vi "HD3000.vi"() -> ()   [LabVIEW 2013]
uses:
  <vilib>/vision/NI_Vision_Development_Module.lvlib
  <vilib>/ptbypt/NI_PtbyPt.lvlib
panel:
  out "Numeric 3":i32
  out "Numeric 2":i32
  out "Numeric":i32
  out "Done":bool caption="Stopped"
  out "error out 4":errorcluster
  out "error out 3":errorcluster
  out "error out 2":errorcluster
  out "Mean Value":sgl
  out "Frame Rate":dbl
  in  "Display":bool
  in  "Rec":bool
  in  "Start":bool
  in  "?":enum32{"Settings", "Monitor", "Errors"}(tab)
  in  "Selected Path for AVI":path
  in  "Cluster":T1={"Brightness"=133, "Contrast"=0.05, "Saturation"=83, "Sharpness"=25, "White Balance"=3040, "Exposure"=0.00048828125, "Auto"=FALSE, "Auto"=FALSE} {"Exposure" min=0.00048828125 max=2.0 scale=0.00048828125..2.0 scale format="%#_1f"; "White Balance" min=2800 max=8000 step=1 scale=2800.0..10000.0; "Sharpness" min=0 max=50 step=1 scale=0.0..50.0; "Saturation" min=0 max=200 step=1 scale=0.0..200.0; "Contrast" min=0.0 max=0.1 scale=0.0..0.1; "Brightness" min=30 max=255 step=1 scale=30.0..255.0}
  out "Rec Time":dbl format="%#_3g"
  out "Est. fps":dbl format="%#_2g"
  out "Frames Recorded":dbl
  out "Frames not Recorded":dbl
  out "Image Number":u32
  out "Lost Image Count":u32
  out "Total Images Transferred":u32
  in  "Interface Name":string="cam1"
  out "error out":errorcluster
  out "Histogram":T2(graph)
  out "Image":T3(plugin-control)
  in  "Stop (F)":bool
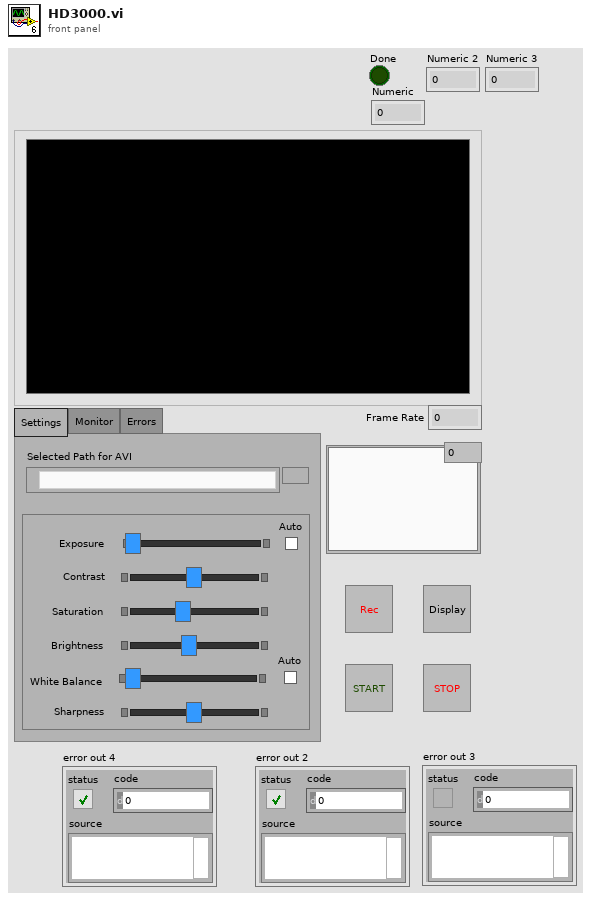
[diagram p1: front panel]
types:
  T1 = cluster{"Brightness":i64, "Contrast":dbl, "Saturation":i64, "Sharpness":i64, "White Balance":i64, "Exposure":dbl, "Auto":bool, "Auto":bool}
  T2 = cluster{"Starting Value":sgl, "Incremental Value":sgl, "Histogram":u32[]}
  T3 = typedef "IMAQ Image.ctl" = refnum<image>
  T4 = typedef "Image Type" = u32
  T5 = typedef "AviRefnum.ctl" = refnum<k1>
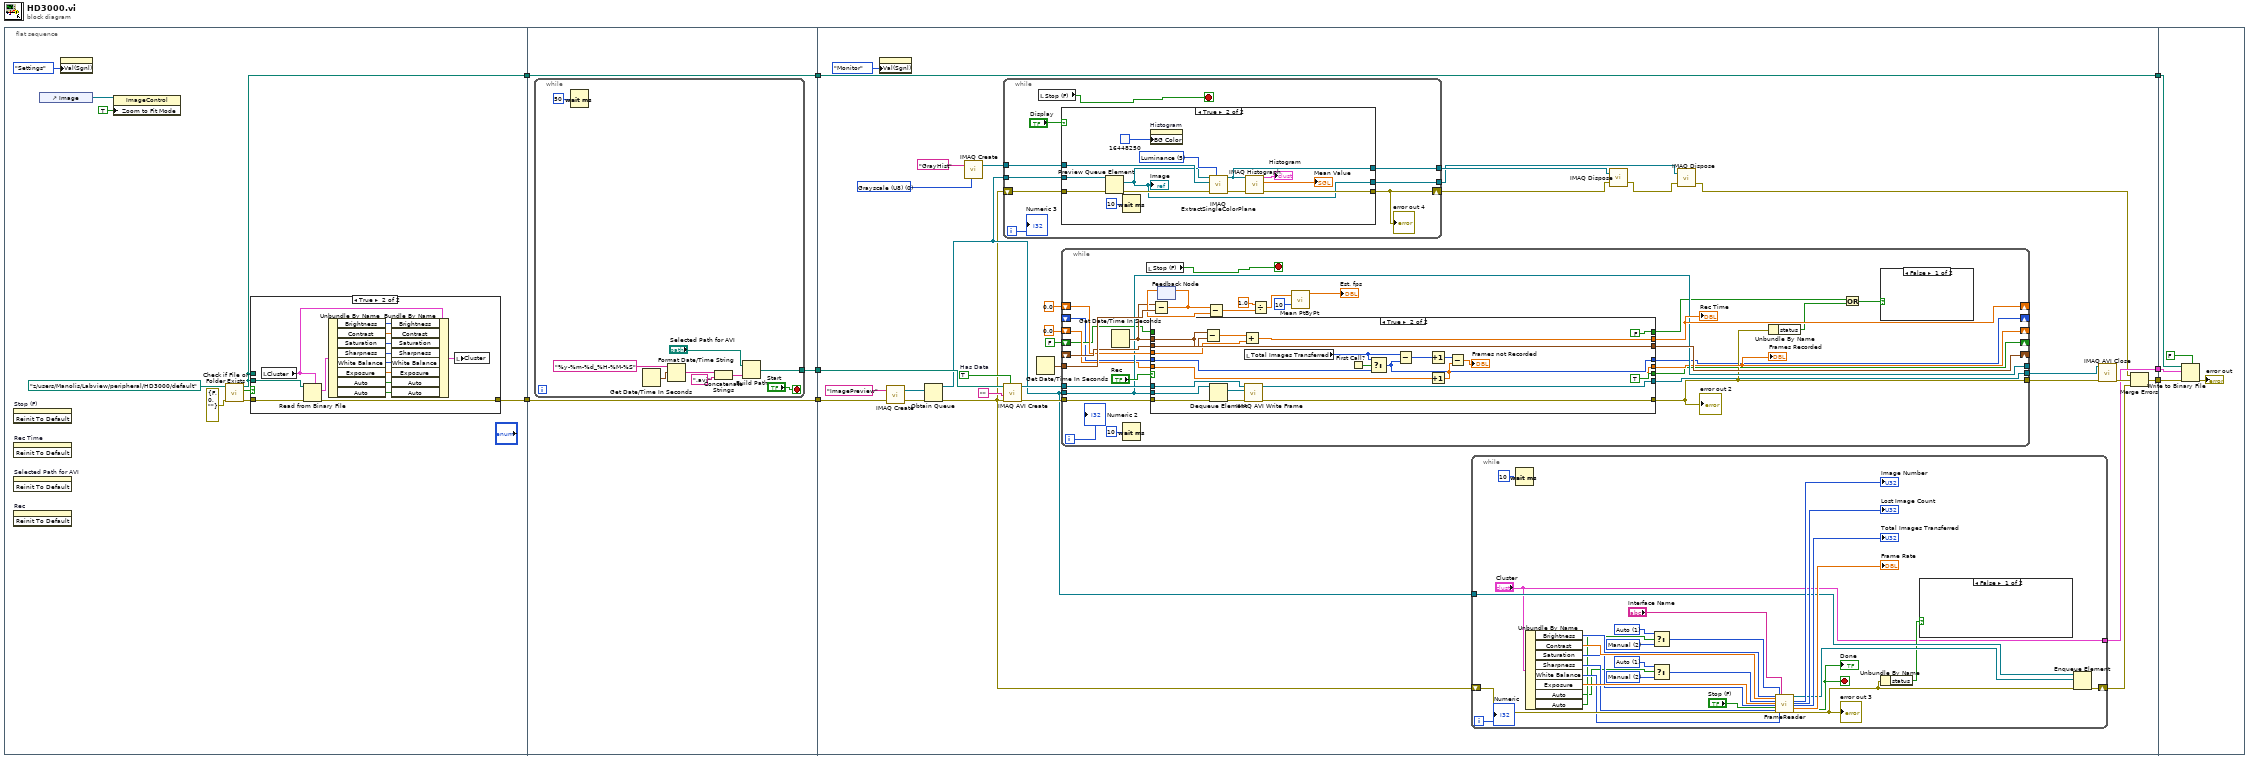
[diagram p0: block diagram]
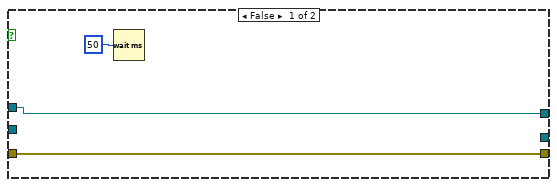
[diagram p3: hidden frame]
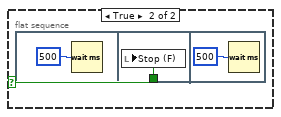
[diagram p4: hidden frame]
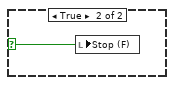
[diagram p5: hidden frame]
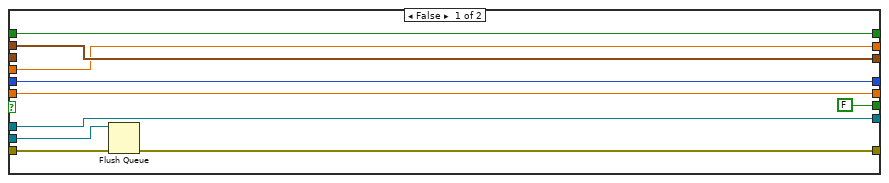
[diagram p6: hidden frame]
diagram:
  n1 = flat-sequence {
    tunnel: [w12] -> w6
    tunnel: [w9] -> w1
    tunnel: [w35] -> w8
    tunnel: w6 -> [w34]
    tunnel: [w34] -> w5
    tunnel: [w33] -> w2
    tunnel: w1 -> [w33]
    tunnel: w8 -> [w71]
    tunnel: [w50] -> w7
    tunnel: w5 -> [w55]
    tunnel: [w55] -> w4
    tunnel: [w54] -> w3
    tunnel: w2 -> [w53]
    tunnel: w7 -> [w204]
    tunnel: w4 -> [w202]
    tunnel: w3 -> [w200]
    frame #0 {
      n2 = invoke on="Stop (F)" class="Bool (strict)" method="Reinit To Default"() -> ()  [unwired: 3 in, 3 out]
      n3 = invoke on="Rec Time" class="DigNum (strict)" method="Reinit To Default"() -> ()  [unwired: 3 in, 3 out]
      n4 = invoke on="Selected Path for AVI" class="Path" method="Reinit To Default"() -> ()  [unwired: 3 in, 3 out]
      n5 = invoke on="Rec" class="Bool (strict)" method="Reinit To Default"() -> ()  [unwired: 3 in, 3 out]
      n6 = control-ref of="Image"() -> (w15:refnum<vi>)
      n7 = property class="TabCtl (strict)"("Val(Sgnl)"=enum32{"Settings", "Monitor"}."Settings" ("Value (Signaling)")) -> ()  [unwired: 2 in, 2 out]
      n8 = property on="Property Node" class="ImageControl"(reference=w15, "Zoom to Fit Mode"=TRUE) -> ()  [unwired: 1 in, 2 out]
      n9 = call <vilib>:"Check if File or Folder Exists.vi"("error in (no error)"=errorcluster {"status"=FALSE, "code"=0, "source"=""} ("error in"), "path"=path "z:/users/Manolis/Labview/peripheral/HD3000/default" ("file path")) -> ("error out"=w10:errorcluster, "file or folder exists?"=w13:bool, "dup path"=w12:path)  [unwired: 7 in]
      n10 = case shown="True" w13 {
        tunnel: w12 -> [_ w23]
        tunnel: w12 -> [_ _]
        tunnel: w10 -> [w18 w22]
        tunnel: [w18 w21] -> w9
        frame False {
        }
        frame True {
          n11 = local read "Cluster"() -> (w20:T1)
          n12 = Read from Binary File(5:w20, 8:w22, 11:w23) -> (0:w21:errorcluster, 2:w32:T1)  [unwired: 3 in, 2 out]
          n13 = Unbundle By Name(w32) -> ("Brightness"=w31:i64, "Contrast"=w30:dbl, "Saturation"=w29:i64, "Sharpness"=w28:i64, "White Balance"=w27:i64, "Exposure"=w26:dbl, "Auto"=w25:bool, "Auto"=w24:bool)
          n14 = Bundle By Name(cluster=w20, "Brightness"=w31, "Contrast"=w30, "Saturation"=w29, "Sharpness"=w28, "White Balance"=w27, "Exposure"=w26, "Auto"=w25, "Auto"=w24) -> (w19:T1)
          n15 = local write "Cluster"(w19) -> ()
        }
      }
    }
    frame #1 {
      n16 = while {
        tunnel: [w36] -> w35
        stop <- "Start" stop-if-true
        n17 = Wait (ms)(milliseconds to wait=u32 50) -> ()  [unwired: 1 out]
        n18 = Get Date/Time In Seconds() -> (seconds since 1Jan1904=w42:timestamp)
        n19 = Format Date/Time String(time format string (%c)="%y-%m-%d_%H-%M-%S", seconds (now)=w42) -> (date/time string=w40:string)  [unwired: 1 in]
        n20 = Concatenate Strings(w40, ".avi" ("search string")) -> (w38:string)
        n21 = Build Path(base path="Selected Path for AVI", name or relative path=w38) -> (appended path=w36:path)
      }
    }
    frame #2 {
      w65 = T4 0 items=["Grayscale (U8)", "Grayscale (I16)", "Grayscale (SGL)", "Complex (CSG)", "RGB (U32)", "HSL (U32)", "RGB (U64)", "Grayscale (U16)"] ("Image Type")
      w67 = TRUE  # Has Data
      n22 = property class="TabCtl (strict)"("Val(Sgnl)"=enum32{"Settings", "Monitor"}."Monitor" ("Value (Signaling)")) -> ()  [unwired: 2 in, 2 out]
      n23 = call "IMAQ Create"("Image Name"="ImagePreview", "error in (no error)"=w53) -> ("New Image"=w61:T3, "error out"=w52:errorcluster)  [unwired: 3 in]
      n24 = Obtain Queue(element data type=w61, error in (no error)=w52) -> (queue out=w60:refnum<queue>, error out=w51:errorcluster)  [unwired: 3 in, 1 out]
      n25 = call "IMAQ Create"("Image Name"="GrayHist", "Image Type"=w65) -> ("New Image"=w63:T3)  [unwired: 3 in, 1 out]
      n26 = while {
        tunnel: w60 -> [w83]
        tunnel: w63 -> [w84]
        shift-right: [w81] -> w48
        shift-left: w51 -> [w80]
        tunnel: [w78] -> w49
        tunnel: [w77] -> w45
        i -> [w79]
        stop <- w76 stop-if-true
        n27 = local read "Stop (F)"() -> (w76:bool)
        n28 = case shown="True" "Display" {
          tunnel: w84 -> [w85 w97]
          tunnel: w83 -> [_ w95]
          tunnel: [w86 w93] -> w81
          tunnel: w80 -> [w86 w92]
          tunnel: [w85 w89] -> w78
          tunnel: [_ w88] -> w77
          frame False {
            n29 = Wait (ms)(milliseconds to wait=u32 50) -> ()  [unwired: 1 out]
          }
          frame True {
            w99 = 5 items=["Red", "Green", "Blue", "Hue", "Saturation", "Luminance", "Value", "Intensity"] ("Color Plane")
            n30 = Preview Queue Element(queue=w95, error in (no error)=w92) -> (element=w88:T3, error out=w91:errorcluster)  [unwired: 1 in, 2 out]
            "Image" <- w88
            n31 = Wait (ms)(milliseconds to wait=u32 10) -> ()  [unwired: 1 out]
            n32 = property on="Histogram" class="WFGraph (strict)"("BG Color"=u32 16448250) -> ()  [unwired: 2 in, 2 out]
            n33 = call "IMAQ ExtractSingleColorPlane"("Color Plane"=w99, "error in (no error)"=w91, "Image Dst"=w97, "Image Src"=w88) -> ("error out"=w94:errorcluster, "Image Dst Out"=w89:T3)  [unwired: 6 in]
            n34 = call "IMAQ Histograph"("error in (no error)"=w94, "Image"=w89) -> ("error out"=w93:errorcluster, "Mean Value"=→"Mean Value":sgl, "Histogram Graph"=→"Histogram":T2)  [unwired: 6 in, 1 out]
          }
        }
        "error out 4" <- w81
        "Numeric 3" <- w79
      }
      n35 = call "IMAQ AVI Create"("Has Data"=w67, "error in (no error)"=w51, "Compression Filter"="", "AVI Path"=w71) -> ("error out"=w72:errorcluster, "Avi Refnum"=w75:T5)  [unwired: 3 in, 3 out]
      n36 = Get Date/Time In Seconds() -> (seconds since 1Jan1904=w69:timestamp)
      n37 = while {
        tunnel: [w165] -> w74
        tunnel: [w145] -> w73
        tunnel: w75 -> [w164]
        tunnel: w72 -> [w163]
        tunnel: w69 -> [w162]
        shift-right: [w161] -> _
        shift-left: _ -> [w160]
        shift-right: [w158] -> _
        shift-left: 0.0 -> [w159]
        tunnel: [w148] -> _
        tunnel: w60 -> [w148]
        shift-right: [w147] -> _
        shift-left: 0.0 -> [w146]
        shift-right: [w144] -> _
        shift-left: FALSE ("First Call?: T/F") -> [w143]
        shift-right: [w140] -> _
        shift-left: _ -> [w139]
        i -> [w136]
        stop <- w135 stop-if-true
        n38 = Get Date/Time In Seconds() -> (seconds since 1Jan1904=w152:timestamp)
        n39 = Wait (ms)(milliseconds to wait=u32 10) -> ()  [unwired: 1 out]
        n40 = local read "Stop (F)"() -> (w135:bool)
        n41 = case shown="True" "Rec" {
          tunnel: [w176 w199] -> w165
          tunnel: [w167 w198] -> w145
          tunnel: w164 -> [w176 w197]
          tunnel: w163 -> [w168 w188]
          tunnel: [w174 w192] -> w158
          tunnel: [w175 w195] -> w161
          tunnel: w152 -> [w175 w195]
          tunnel: w160 -> [_ w194]
          tunnel: w159 -> [w174 w193]
          tunnel: w148 -> [w173 w191]
          tunnel: [w172 w178] -> w147
          tunnel: w146 -> [w172 w189]
          tunnel: [FALSE ("First Call?: T/F") TRUE ("First Call?: T/F")] -> w144
          tunnel: w143 -> [w171 _]
          tunnel: [w171 FALSE ("First Call?: T/F")] -> w142
          tunnel: [w169 w182] -> w140
          tunnel: w139 -> [w169 w183]
          frame False {
            n42 = Flush Queue(queue=w173, error in (no error)=w168) -> (error out=w167:errorcluster)  [unwired: 2 out]
          }
          frame True {
            n43 = Subtract(x=w195, y=w194) -> (x-y=w196:dbl)
            n44 = Dequeue Element(queue=w191, error in (no error)=w188) -> (element=w190:T3, error out=w187:errorcluster)  [unwired: 1 in, 2 out]
            n45 = Add(x=w196, y=w193) -> (x+y=w192:dbl)
            n46 = local read "Total Images Transferred"() -> (w181:u32)
            n47 = call "IMAQ AVI Write Frame"("error in (no error)"=w187, "Image"=w190, "Avi Refnum"=w197) -> ("error out"=w198:errorcluster, "Avi Refnum (duplicate)"=w199:T5)  [unwired: 7 in]
            n48 = First Call?() -> (First Call?: T/F=w184:bool)
            n49 = Select(t=w181, s=w184, f=w183) -> (s? t:f=w182:u32)
            n50 = Subtract(x=w181, y=w182) -> (x-y=w180:u32)
            n51 = Increment(x=w180) -> (x+1=w179:u32)
            n52 = Increment(x=w189) -> (x+1=w178:dbl)
            n53 = Subtract(x=w179, y=w178) -> (x-y=→"Frames not Recorded":dbl)
          }
        }
        "Rec Time" <- w158
        "Frames Recorded" <- w147
        "error out 2" <- w145
        n54 = Subtract(x=w152, y=w162) -> (x-y=w153:dbl)
        n55 = feedback #1() -> (w157:dbl)  [unwired: 1 in]
        n56 = feedback-in #1(w153) -> ()
        n57 = Subtract(x=w153, y=w157) -> (x-y=w155:dbl)
        n58 = Divide(x=1.0, y=w155) -> (x/y=w154:dbl)
        n59 = call <vilib>:"Mean PtByPt.vi"("x"=w154, "sample length"=10) -> ("mean"=→"Est. fps":dbl)  [unwired: 2 in, 1 out]
        n60 = Unbundle By Name(w145) -> ("status"=w141:bool)
        n61 = Or(x=w142, y=w141) -> (x .or. y?=w138:bool)
        n62 = case shown="False" w138 {
          selector: w138 -> [_ w166]
          frame False {
          }
          frame True {
            n63 = local write "Stop (F)"(w166) -> ()
          }
        }
        "Numeric 2" <- w136
      }
      n64 = while {
        tunnel: w60 -> [w124]
        shift-right: [w115] -> w57
        shift-left: w51 -> [w117]
        tunnel: ["Cluster"] -> w50
        i -> [w101]
        stop <- w113 stop-if-true
        w118 = u32 2 items=["Auto"=1, "Manual"=2] ("Exposure::Mode")
        w119 = u32 1 items=["Auto"=1, "Manual"=2] ("Exposure::Mode")
        w122 = u32 2 items=["Auto"=1, "Manual"=2] ("Exposure::Mode")
        w123 = u32 1 items=["Auto"=1, "Manual"=2] ("Exposure::Mode")
        n65 = Wait (ms)(milliseconds to wait=u32 10) -> ()  [unwired: 1 out]
        n66 = Unbundle By Name("Cluster") -> ("Brightness"=w111:i64, "Contrast"=w110:dbl, "Saturation"=w108:i64, "Sharpness"=w107:i64, "White Balance"=w106:i64, "Exposure"=w109:dbl, "Auto"=w103:bool, "Auto"=w104:bool)
        n67 = Select(t=w119, s=w104, f=w118) -> (s? t:f=w120:u32)
        n68 = Select(t=w123, s=w103, f=w122) -> (s? t:f=w121:u32)
        n69 = call "FrameReader.vi"("Brightness::Value"=w111, "Contrast::Value"=w110, "Exposure::Mode"=w121, "Exposure::Value"=w109, "Saturation::Value"=w108, "Stop (F)"="Stop (F)", "Sharpness::Value"=w107, "error in"=w117, "White Balance::Mode"=w120, "White Balance::Value"=w106, "Interface Name"="Interface Name") -> ("Image Out"=w125:T3, "Image Number"=→"Image Number":u32, "Lost Image Count"=→"Lost Image Count":u32, "Total Images Transferred"=→"Total Images Transferred":u32, "Frame Rate"=→"Frame Rate":dbl, "Stopped"=w113:bool, "error out"=w116:errorcluster)  [unwired: 9 in, 1 out]
        "error out 3" <- w116
        "Done" <- w113
        n70 = Unbundle By Name(w116) -> ("status"=w114:bool)
        n71 = case shown="False" w114 {
          selector: w114 -> [_ w131]
          frame False {
          }
          frame True {
            n72 = flat-sequence {
              tunnel: w131 -> [w133]
              frame #0 {
                n73 = Wait (ms)(milliseconds to wait=u32 500) -> ()  [unwired: 1 out]
              }
              frame #1 {
                n74 = local write "Stop (F)"(w133) -> ()
              }
              frame #2 {
                n75 = Wait (ms)(milliseconds to wait=u32 500) -> ()  [unwired: 1 out]
              }
            }
          }
        }
        n76 = Enqueue Element(queue=w124, element=w125, error in (no error)=w116) -> (error out=w115:errorcluster)  [unwired: 1 in, 2 out]
        "Numeric" <- w101
      }
      n77 = call "IMAQ Dispose"("Image"=w49, "error in (no error)"=w48) -> ("error out"=w47:errorcluster)  [unwired: 4 in]
      n78 = call "IMAQ Dispose"("Image"=w45, "error in (no error)"=w47) -> ("error out"=w46:errorcluster)  [unwired: 4 in]
      n79 = call "IMAQ AVI Close"("error in (no error)"=w73, "Avi Refnum"=w74) -> ("error out"=w58:errorcluster)  [unwired: 9 in]
      n80 = Merge Errors(w46, w58, w57) -> (w54:errorcluster)
    }
    frame #3 {
      n81 = Write to Binary File(file (use dialog)=w202, data=w204, error in=w200, 5:FALSE ("prepend array or string size? (T)")) -> (error out=→"error out":errorcluster)  [unwired: 2 in, 2 out]
    }
  }
